vi "LVClass_Image Is processed image.vi"(0 "Image in":refnum<class "Image.lvclass">, 11 "error in (no error)":errorcluster) -> (4 "Image out":refnum<class "Image.lvclass">, 6 "background_removed":bool, 8 "filtered_image_removed":bool, 15 "error out":errorcluster)   [LabVIEW 2020, in "Image.lvclass"]
doc: "Get metadata from Image object.\n\n--------------------------------------------------------------------------------\n\n<B>ImageIn </B> : Image object.\n<B>ImageOut </B> : Image object.\n<B>haso_serial_number </B> : Haso serial number.\n<B>camera_serial_number </B> : Camera serial number.\n<B>exposure_time_applied </B> : Exposure duration applied (us).\n<B>exposure_time_requested </B> : Exposure duration requested (us).\n<B>gain </B> : Applied gain (SI).\n<B>nb_summed_images </B> : Number of summed images.\n<B>is_smearing_removed </B> : Smearing_removed.\n<B>is_background_removed </B> : Background_removed.\n<B>trigger_type </B> : Trigger mode.\n<B>time_stamp </B> : Date of the acquired Image.\n<B>max_level </B> : Max level value.\n<B>comments </B> : Comments.\n<B>ErrorIn </B> : Error\n<B>ErrorOut </B> : Error\n\n--------------------------------------------------------------------------------"
uses:
  Image.lvclass
  Image.lvclass/Image.ctl
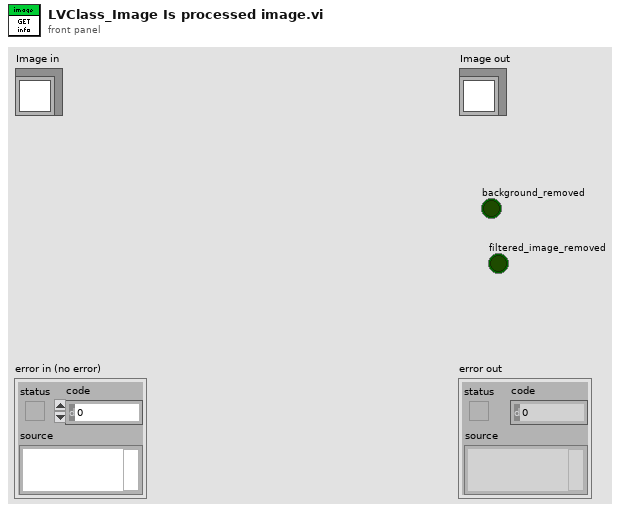
[diagram p1: front panel]
types:
  T1 = typedef "ClassID.ctl" = i64
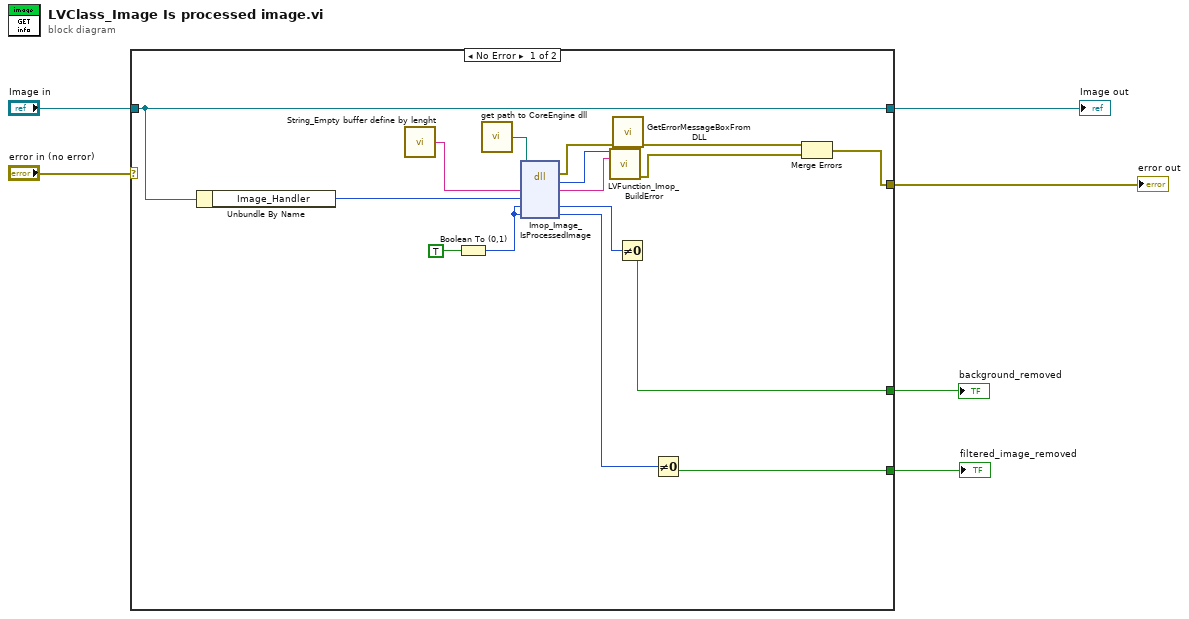
[diagram p0: block diagram]
diagram:
  n1 = case shown="No Error" "error in (no error)" {
    selector: "error in (no error)" -> [_ w24]
    tunnel: [w13 w24] -> w5
    tunnel: [w11 w23] -> w3
    tunnel: "Image in" -> [w11 w23]
    tunnel: [w10 _] -> w2
    tunnel: [w7 _] -> w1
    frame No Error {
      n2 = Unbundle By Name(w11) -> ("Image_Handler"=w22:T1)
      n3 = call "String_Empty buffer define by lenght.vi"() -> ("Empty buffer"=w12:string)  [unwired: 1 in]
      n4 = Boolean To (0,1)(Boolean=TRUE) -> (0, 1=w9:i16)
      n5 = call "get path to CoreEngine dll.vi"() -> ("path to wavekit library"=w19:path)  [unwired: 14 in, 1 out]
      n6 = dll-call lib="D:/2_trunk/Soft_haso/ImOpCoreEngine4_LV2011/DLLs/ImopEngine4_vc100.dll" fn="Imop_Image_IsProcessedImage"(path in=w19, "message"=w12, "Image compat"=w22, "background_removed"=w9, "filtered_image_removed"=w9) -> (error out=w18:errorcluster, "return type"=w21:i32, "message"=w20:string, "background_removed"=w16:u8, "filtered_image_removed"=w8:u8)  [unwired: 3 in, 1 out]
      n7 = call "LVFunction_Imop_BuildError.vi"("code"=w21, "String to Prepend to source (\"\")"=w20) -> ("error out"=w14:errorcluster)  [unwired: 13 in]
      n8 = call "GetErrorMessageBoxFromDLL.vi"("error IN"=w18) -> ("error OUT"=w15:errorcluster)  [unwired: 10 in]
      n9 = Not Equal To 0?(x=w16) -> (x != 0?=w10:bool)
      n10 = Not Equal To 0?(x=w8) -> (x != 0?=w7:bool)
      n11 = Merge Errors(w15, w14) -> (w13:errorcluster)
    }
    frame Error {
    }
  }
  "error out" <- w5
  "Image out" <- w3
  "background_removed" <- w2
  "filtered_image_removed" <- w1
